vi "Moving Average (single).vi"(8 "error in (no error)":errorcluster, 10 "window":dbl, 11 "XY-data":cluster{"X-array":dbl[], "Y-array":dbl[]}) -> (0 "error out":errorcluster, 3 "XY-data out":cluster{"X-array":dbl[], "Y-array":dbl[]} {"Y-array" format="%.2p"; "X-array" format="%.2p"})   [LabVIEW 2016, in "xy_utilities.lvlib"]
doc: "Apply a moving average <b>XY-data</b>'s Y-Array according to <b>window</b>\n\nWire data to the data input to determine the polymorphic instance to use or manually select the instance."
uses:
  xy_utilities.lvlib
  <vilib>/ptbypt/NI_PtbyPt.lvlib
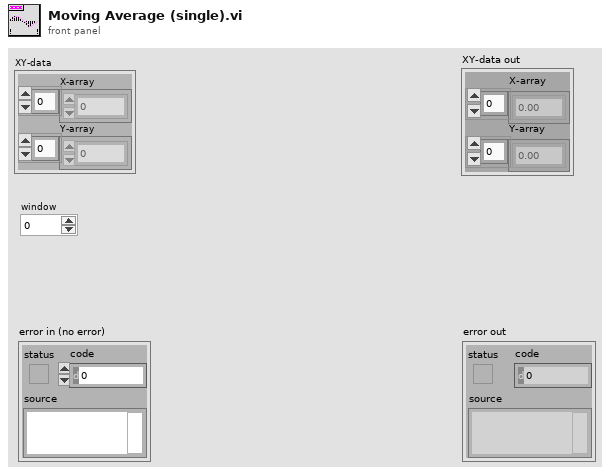
[diagram p1: front panel]
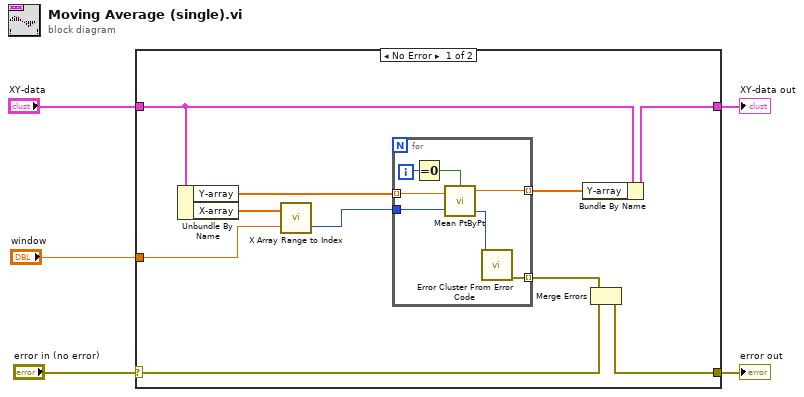
[diagram p0: block diagram]
diagram:
  n1 = case shown="No Error" "error in (no error)" {
    selector: "error in (no error)" -> [w8 w24]
    tunnel: [w7 w24] -> w4
    tunnel: "XY-data" -> [w12 w23]
    tunnel: [w15 w23] -> w2
    tunnel: "window" -> [w11 _]
    frame No Error {
      n2 = Unbundle By Name(w12) -> ("Y-array"=w14:dbl[], "X-array"=w10:dbl[])
      n3 = call "X Array Range to Index.vi"("X Range"=w11, "X-array"=w10) -> ("X Range (index)"=w6:i32)  [unwired: 1 in]
      n4 = for {
        tunnel: w14 -> [w22] mode=indexing
        tunnel: [w21] -> w13 mode=indexing
        tunnel: w6 -> [w20]
        tunnel: [w16] -> w9 mode=indexing
        i -> [w18]
        n5 = Equal To 0?(x=w18) -> (x = 0?=w19:bool)
        n6 = call <vilib>:"Mean PtByPt.vi"("x"=w22, "sample length"=w20, "initialize"=w19) -> ("mean"=w21:dbl, "error"=w17:i32)  [unwired: 1 in]
        n7 = call <vilib>:"Error Cluster From Error Code.vi"("error code (0)"=w17) -> ("error out"=w16:errorcluster)  [unwired: 8 in]
      }
      n8 = Bundle By Name(cluster=w12, "Y-array"=w13) -> (w15:cluster{"X-array":dbl[], "Y-array":dbl[]})
      n9 = Merge Errors(w9, w8) -> (w7:errorcluster)
    }
    frame Error {
    }
  }
  "error out" <- w4
  "XY-data out" <- w2
